vi "Test.UDP.vi"() -> ()   [LabVIEW 2014]
panel:
  out "Now (us)":dbl=1.0 format="%.2f"
  in  "Parameter":u16(ring) items=["Frequency (MHz)", "Amplitude (dBm)", "Phase (Pi)"]
  in  "Start":dbl=1.0 format="%.3f"
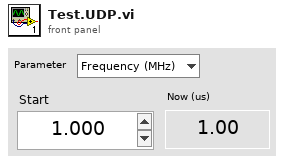
[diagram p1: front panel]
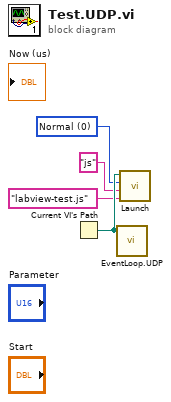
[diagram p0: block diagram]
diagram:
  w1 = u16 0 items=["Normal", "Keep", "Hide"] ("Mode")
  n1 = Current VI's Path() -> (path=w4:path)
  n2 = call "EventLoop.UDP.vi"("Path"=w4) -> ()  [unwired: 2 in]
  n3 = call "Launch.vi"("File"="labview-test.js", "Cmd"="js", "Mode"=w1, "Path"=w4) -> ()
